vi "Log Error.vi"(8 "Error In":errorcluster) -> (0 "Error Out":errorcluster)   [LabVIEW 2012]
uses:
  <userlib>/Library.lnk/File IO/Path Operations/Application Folder Paths Option.ctl
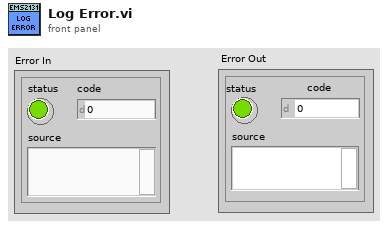
[diagram p1: front panel]
types:
  T1 = typedef "Application Folder Paths Option.ctl" = enum16{"Application Files", "Binary Files", "Configuration Files", "Log Files", "Report Files", "Dictionaries"}
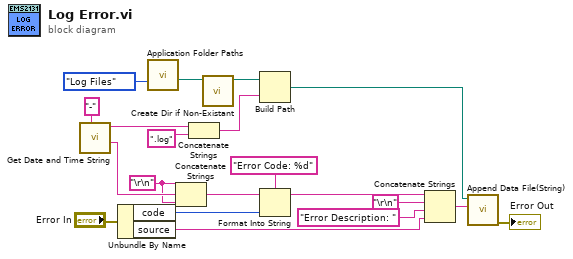
[diagram p0: block diagram]
diagram:
  w1 = "\r\n"
  n1 = call <userlib>:"Get Date and Time String.vi"("Seperator"="-") -> ("Time"=w2:string, "Date"=w17:string)  [unwired: 3 in, 6 out]
  n2 = Unbundle By Name("Error In") -> ("code"=w11:i32, "source"=w9:string)
  n3 = call <userlib>:"Application Folder Paths.vi"("Path Option"=Application_Folder_Paths_Option."Log Files") -> ("Path"=w16:path)  [unwired: 1 in, 9 out]
  n4 = Concatenate Strings(w1, w2, w1) -> (w4:string)
  n5 = Concatenate Strings(w17, ".log" ("string")) -> (w14:string)
  n6 = call <userlib>:"Create Dir if Non-Existant.vi"("Directory Path"=w16) -> ("dup Directory Path"=w18:path)  [unwired: 2 in, 8 out]
  n7 = Build Path(base path=w18, name or relative path=w14) -> (appended path=w12:path)
  n8 = Format Into String(format string="Error Code: %d", initial string=w4, w11) -> (resulting string=w10:string)  [unwired: 1 in, 1 out]
  n9 = Concatenate Strings(w10, "\r\n", "Error Description: " ("string"), w9) -> (w8:string)
  n10 = call <userlib>:"Append Data File(String).vi"("Data"=w8, "File path"=w12) -> ("error out"=→"Error Out":errorcluster)  [unwired: 9 in]
